vi "Call Client Generator.vi"(8 "error in":errorcluster, 11 "generation data":T1) -> (0 "error out":errorcluster)   [LabVIEW 2024, in "gRPC Client Generation.lvlib"]
uses:
  gRPC Client Generation.lvlib
  Generation Data.ctl
  <vilib>/gRPC/gRPC Server and Client Template [2]/gRPC Scripting Tools/Main.vi
  <vilib>/gRPC/gRPC Server and Client Template [2]/gRPC Scripting Tools/gRPC Template Creation Utility-release.lvlib
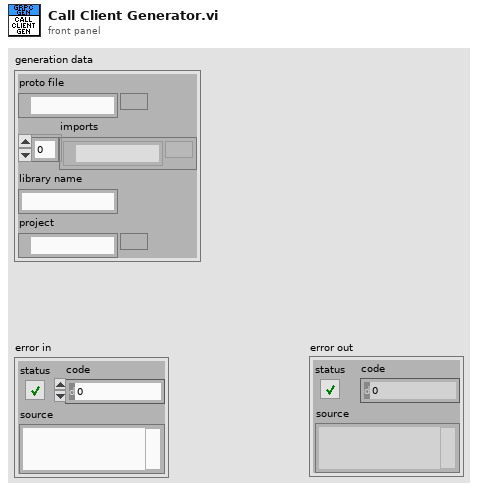
[diagram p1: front panel]
types:
  T1 = typedef "gRPC Client Generation.lvlib/Generation Data.ctl" = cluster{"proto file":path, "imports":path[], "library name":string, "project":path}
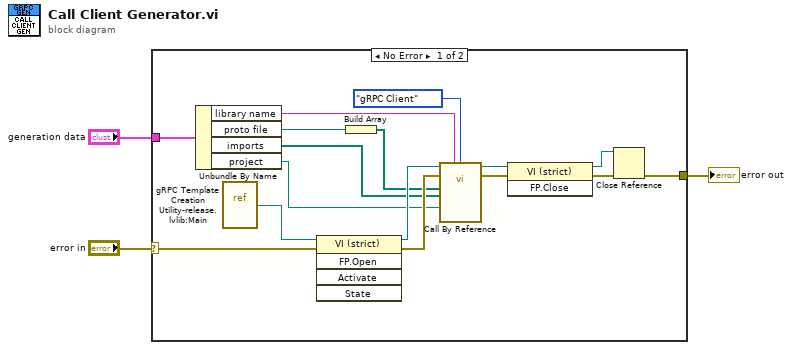
[diagram p0: block diagram]
diagram:
  n1 = case shown="No Error" "error in" {
    selector: "error in" -> [w4 w20]
    tunnel: "generation data" -> [w11 _]
    tunnel: [w5 w20] -> w2
    frame No Error {
      n2 = Unbundle By Name(w11) -> ("library name"=w6:string, "proto file"=w10:path, "imports"=w8:path[], "project"=w7:path)
      n3 = vi-ref "gRPC Template Creation Utility-release.lvlib:Main.vi"() -> (w16:refnum<vi>)
      n4 = invoke class="VI (strict)" method="FP.Open"(reference=w16, error in=w4) -> (reference out=w18:refnum<vi>, error out=w17:errorcluster)  [unwired: 3 in, 3 out]
      n5 = Build Array(w10) -> (w9:path[])
      n6 = call-by-ref "?"(reference=w18, error in=w17, "Proto File Path"=w9, "Generated Library Name"=w6, "Generate"=enum16{"gRPC Server", "gRPC Client", "Both"}."gRPC Client", "Import Paths"=w8, "Target Project"=w7) -> (reference out=w15:refnum<vi>, error out=w14:errorcluster)  [unwired: 11 in]
      n7 = invoke class="VI (strict)" method="FP.Close"(reference=w15, error in=w14) -> (reference out=w13:refnum<vi>, error out=w12:errorcluster)  [unwired: 1 in, 1 out]
      n8 = Close Reference(reference=w13, error in (no error)=w12) -> (error out=w5:errorcluster)
    }
    frame Error {
    }
  }
  "error out" <- w2
